vi "request file path.vi"(8 "error in (no error)":errorcluster, 11 "data log in":refnum<class "data log.lvclass">) -> (0 "error out":errorcluster, 2 "selected path":path, 3 "data log out":refnum<class "data log.lvclass">)   [LabVIEW 2025, in "data log.lvclass"]
uses:
  data log.lvclass
  <vilib>/Utility/sysdir.llb/System Directory Type.ctl
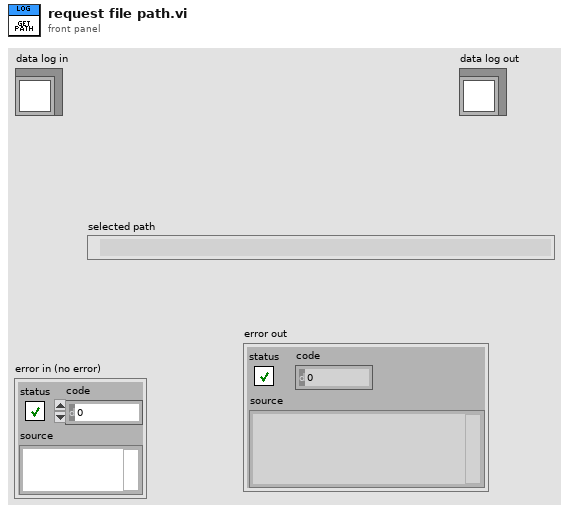
[diagram p1: front panel]
types:
  T1 = typedef "System Directory Type.ctl" = i32
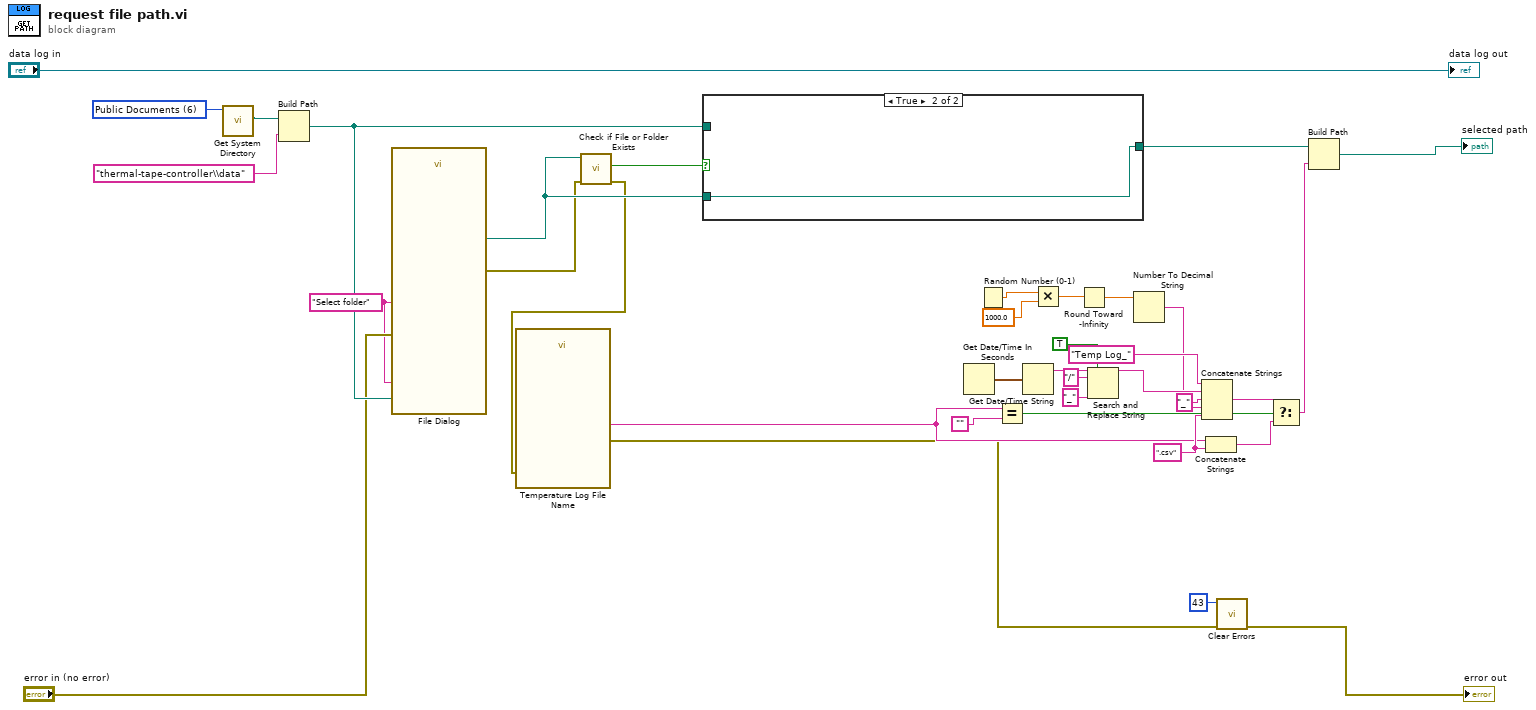
[diagram p0: block diagram]
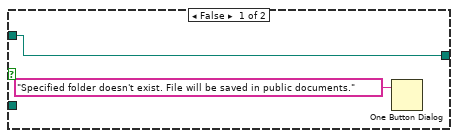
[diagram p2: hidden frame]
diagram:
  w7 = ".csv" ("string")
  w1 = "Select folder" ("button label")
  w33 = T1 6 items=["User Home"=0, "User Desktop"=1, "User Documents"=2, "User Application Data"=3, "User Preferences"=4, "User Temporary"=5, "Public Documents"=6, "Public Application Data"=7, "Public Preferences"=8, "Public Cache"=13, "System Core Libraries"=9, "System Installed Libraries"=10, "Application Files"=11, "Boot Volume Root"=12] ("system directory type")
  n1 = call <vilib>:"Get System Directory.vi"("system directory type"=w33) -> ("system directory"=w32:path)  [unwired: 10 in]
  n2 = Build Path(base path=w32, name or relative path="thermal-tape-controller\\data") -> (appended path=w13:path)
  n3 = call "File Dialog"("start path"=w13, "prompt"=w1, "button label"=w1, "error in"="error in (no error)") -> ("selected path"=w12:path, "error out"=w11:errorcluster)  [unwired: 8 in, 2 out]
  n4 = call <vilib>:"Check if File or Folder Exists.vi"("error in (no error)"=w11, "path"=w12) -> ("error out"=w10:errorcluster, "file or folder exists?"=w14:bool)  [unwired: 7 in, 1 out]
  n5 = call "Temperature Log File Name"("error in (no error)"=w10) -> ("File name"=w6:string, "error out"=w3:errorcluster)  [unwired: 16 in, 1 out]
  n6 = case shown="True" w14 {
    tunnel: [w37 w39] -> w9
    tunnel: w13 -> [w37 _]
    tunnel: w12 -> [_ w39]
    frame False {
      n7 = One Button Dialog(message="Specified folder doesn't exist. File will be saved in public documents.") -> ()  [unwired: 1 in, 1 out]
    }
    frame True {
    }
  }
  n8 = Get Date/Time In Seconds() -> (seconds since 1Jan1904=w28:timestamp)
  n9 = Random Number (0-1)() -> (number: 0 to 1=w20:dbl)
  n10 = Equal?(x=w6, y="") -> (x = y?=w29:bool)
  n11 = Get Date/Time String(seconds (now)=w28) -> (date string=w27:string)  [unwired: 2 in, 1 out]
  n12 = Multiply(x=w20, y=1000.0) -> (x*y=w18:dbl)
  n13 = Round Toward -Infinity(1:w18) -> (0:w17:dbl)
  n14 = Search and Replace String(replace all?=TRUE ("replace all? (F)"), input string=w27, search string="/", replace string="_" ("replace string (\"\")")) -> (result string=w24:string)  [unwired: 4 in, 3 out]
  n15 = Number To Decimal String(number=w17) -> (decimal integer string=w16:string)  [unwired: 1 in]
  n16 = Concatenate Strings("Temp Log_" ("string"), w24, "_" ("string"), w16, w7) -> (w22:string)
  n17 = Concatenate Strings(w6, w7) -> (w5:string)
  n18 = call <vilib>:"Clear Errors.vi"("error in (no error)"=w3, "specific error code to clear (0: all)"=43) -> ("error out"=→"error out":errorcluster)  [unwired: 4 in, 1 out]
  n19 = Select(t=w22, s=w29, f=w5) -> (s? t:f=w8:string)
  n20 = Build Path(base path=w9, name or relative path=w8) -> (appended path=→"selected path":path)
  "data log out" <- "data log in"
